vi "Get All RTMs from Project.vi"(8 "error in (no error)":errorcluster, 11 "Project Path":path) -> (0 "error out":errorcluster, 2 "RTM Virtual Paths":string[](array[string]), 3 "Project RTMs":path[](array[path]), 5 "Project Name":string)   [LabVIEW 2013, in "SET Project Editor.lvlib"]
doc: "Get All RTMs from Project.vi\n\nReturns paths (relative to project root) and virtual paths to all\nRTM files included in the LabVIEW project."
uses:
  SET Project Editor.lvlib
panel:
  # "Get All RTMs from Project.vi\n\nReturns paths (relative to project root) and virtual paths to all\nRTM files included in the LabVIEW project."
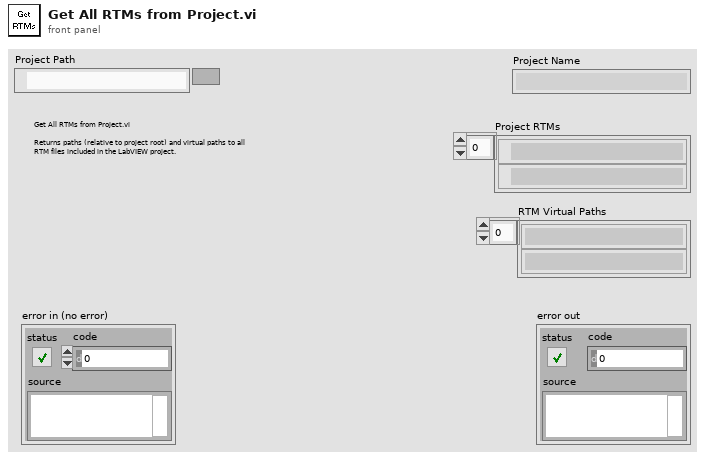
[diagram p1: front panel]
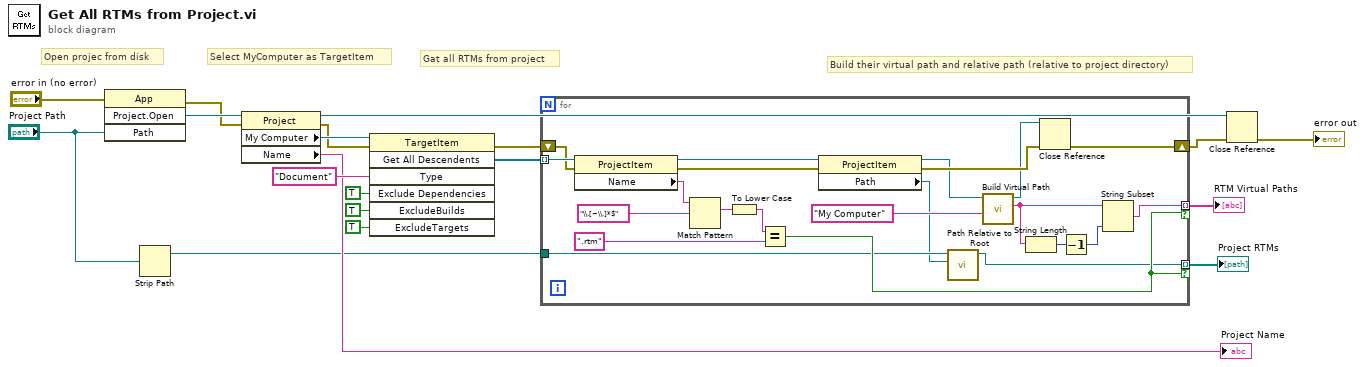
[diagram p0: block diagram]
diagram:
  # "Build their virtual path and relative path (relative to project directory)"
  # "Gat all RTMs from project"
  # "Select MyComputer as TargetItem"
  # "Open projec from disk"
  n1 = invoke class="App" method="Project.Open"(error in="error in (no error)", "Path"="Project Path") -> (error out=w12:errorcluster, "Project:Open"=w15:refnum<vi>)  [unwired: 2 in, 2 out]
  n2 = Strip Path(path="Project Path") -> (stripped path=w3:path)  [unwired: 1 out]
  n3 = property class="Project"(reference=w15, error in=w12) -> (reference out=w6:refnum<vi>, error out=w11:errorcluster, "My Computer"=w14:refnum<vi>, "Name"=→"Project Name":string)
  n4 = invoke class="TargetItem" method="Get All Descendents"(reference=w14, error in=w11, "Type"="Document", "Exclude Dependencies"=TRUE ("ExcludeDependencies"), "ExcludeBuilds"=TRUE, "ExcludeTargets"=TRUE) -> (error out=w9:errorcluster, "All Descendents"=w10:refnum<vi>[])  [unwired: 1 in, 5 out]
  n5 = for {
    tunnel: w10 -> [w32] mode=indexing
    shift-right: [w41] -> w7
    shift-left: w9 -> [w30]
    tunnel: w3 -> [w22]
    tunnel: [w20] -> w2 mode=indexing if=w28
    tunnel: [w33] -> w1 mode=indexing if=w28
    n6 = property class="ProjectItem"(reference=w32, error in=w30) -> (reference out=w31:refnum<vi>, error out=w29:errorcluster, "Name"=w25:string)
    n7 = Match Pattern(string=w25, regular expression="\\.[~\\.]*$") -> (match substring=w23:string)  [unwired: 4 out]
    n8 = To Lower Case(string=w23) -> (all lower case string=w24:string)
    n9 = Equal?(x=w24, y=".rtm") -> (x = y?=w28:bool)
    n10 = property class="ProjectItem"(reference=w31, error in=w29) -> (reference out=w39:refnum<vi>, error out=w40:errorcluster, "Path"=w21:path)
    n11 = call "Path Relative to Root.vi"("ItemPath"=w21, "RootDir"=w22) -> ("ItemPath (Relative to Root)"=w20:path)  [unwired: 9 in]
    n12 = call "Build Virtual Path.vi"("ProjItem* in"=w39, "Top Level Name"="My Computer") -> ("ProjItem* out"=w38:refnum<vi>, "VI ProjPath out"=w34:string)  [unwired: 6 in, 1 out]
    n13 = String Length(string=w34) -> (length=w36:i32)
    n14 = Close Reference(reference=w38, error in (no error)=w40) -> (error out=w41:errorcluster)
    n15 = Decrement(x=w36) -> (x-1=w35:i32)
    n16 = String Subset(string=w34, length (rest)=w35) -> (substring=w33:string)  [unwired: 1 in]
  }
  "Project RTMs" <- w2
  "RTM Virtual Paths" <- w1
  n17 = Close Reference(reference=w6, error in (no error)=w7) -> (error out=→"error out":errorcluster)
